vi "RTS Set Test Start Time.vi"(4 "Use Current Time As Start?":bool, 5 "Time Start (Gen Prev End)":timestamp, 6 "index":i32, 7 "Start Time Offset":dbl, 8 "Error In":errorcluster, 11 "Current Test":T1={"Chamber 1-3"=[{"End Time"=timestamp(3594046716.8947463 s since 1904-01-01), "Start Time"=timestamp(3593614713.19836 s since 1904-01-01), "Door Opening Schedule:"={"Open Door Timer (s)"=12.0, "Delay Time (s)"=695.0, "Close Door Timer (s)"=12.0}, "Enable Door Ops"=TRUE, "Door Openings"=120, "Temp (°F)"=0.0, "Humidity (%)"=0.0, "Voltage (V)"=0.0, "Door Open Sequence:"=enum."", "Door Delay(sec)"=0.0, "Dehum (°F)"=0.0, "Cool (°F)"=0.0}], "Chamber 1-2"=[{"End Time"=timestamp(3594046708.565822 s since 1904-01-01), "Start Time"=timestamp(3593614700.612354 s since 1904-01-01), "Door Opening Schedule:"={"Open Door Timer (s)"=12.0, "Delay Time (s)"=695.0, "Close Door Timer (s)"=12.0}, "Enable Door Ops"=TRUE, "Door Openings"=0, "Temp (°F)"=0.0, "Humidity (%)"=0.0, "Voltage (V)"=0.0, "Door Open Sequence:"=enum."", "Door Delay(sec)"=0.0, "Dehum (°F)"=0.0, "Cool (°F)"=0.0}], "Chamber 1-1"=[{"End Time"=timestamp(3594046691.867131 s since 1904-01-01), "Start Time"=timestamp(3593614687.850203 s since 1904-01-01), "Door Opening Schedule:"={"Open Door Timer (s)"=12.0, "Delay Time (s)"=2800.0, "Close Door Timer (s)"=12.0}, "Enable Door Ops"=TRUE, "Door Openings"=30, "Temp (°F)"=0.0, "Humidity (%)"=0.0, "Voltage (V)"=0.0, "Door Open Sequence:"=enum."", "Door Delay(sec)"=0.0, "Dehum (°F)"=0.0, "Cool (°F)"=0.0}], "Standard Tests 1-1"=enum."511-B111 Internal Moisture"} {"Chamber 1-1"."Start Time" format="%<%X\n%x>T"; "Chamber 1-1"."End Time" format="%<%X\n%x>T"; "Chamber 1-2"."Start Time" format="%<%X\n%x>T"; "Chamber 1-2"."End Time" format="%<%X\n%x>T"; "Chamber 1-3"."Start Time" format="%<%X\n%x>T"; "Chamber 1-3"."End Time" format="%<%X\n%x>T"}) -> (0 "Error Out":errorcluster, 3 "Current Test Output":T1={"Chamber 1-3"=[{"End Time"=timestamp(3594046716.8947463 s since 1904-01-01), "Start Time"=timestamp(3593614713.19836 s since 1904-01-01), "Door Opening Schedule:"={"Open Door Timer (s)"=12.0, "Delay Time (s)"=695.0, "Close Door Timer (s)"=12.0}, "Enable Door Ops"=TRUE, "Door Openings"=120, "Temp (°F)"=0.0, "Humidity (%)"=0.0, "Voltage (V)"=0.0, "Door Open Sequence:"=enum."", "Door Delay(sec)"=0.0, "Dehum (°F)"=0.0, "Cool (°F)"=0.0}], "Chamber 1-2"=[{"End Time"=timestamp(3594046708.565822 s since 1904-01-01), "Start Time"=timestamp(3593614700.612354 s since 1904-01-01), "Door Opening Schedule:"={"Open Door Timer (s)"=12.0, "Delay Time (s)"=695.0, "Close Door Timer (s)"=12.0}, "Enable Door Ops"=TRUE, "Door Openings"=0, "Temp (°F)"=0.0, "Humidity (%)"=0.0, "Voltage (V)"=0.0, "Door Open Sequence:"=enum."", "Door Delay(sec)"=0.0, "Dehum (°F)"=0.0, "Cool (°F)"=0.0}], "Chamber 1-1"=[{"End Time"=timestamp(3594046691.867131 s since 1904-01-01), "Start Time"=timestamp(3593614687.850203 s since 1904-01-01), "Door Opening Schedule:"={"Open Door Timer (s)"=12.0, "Delay Time (s)"=2800.0, "Close Door Timer (s)"=12.0}, "Enable Door Ops"=TRUE, "Door Openings"=30, "Temp (°F)"=0.0, "Humidity (%)"=0.0, "Voltage (V)"=0.0, "Door Open Sequence:"=enum."", "Door Delay(sec)"=0.0, "Dehum (°F)"=0.0, "Cool (°F)"=0.0}], "Standard Tests 1-1"=enum."511-B111 Internal Moisture"} {"Chamber 1-1"."Start Time" format="%<%X\n%x>T"; "Chamber 1-1"."End Time" format="%<%X\n%x>T"; "Chamber 1-2"."Start Time" format="%<%X\n%x>T"; "Chamber 1-2"."End Time" format="%<%X\n%x>T"; "Chamber 1-3"."Start Time" format="%<%X\n%x>T"; "Chamber 1-3"."End Time" format="%<%X\n%x>T"})   [LabVIEW 2020]
uses:
  Type Definitions/RTS Door Op Data.ctl
  Type Definitions/RTS Door Ops Client.ctl
  Type Definitions/RTS Door Opening Schedule.ctl
  Type Definitions/RTS Door Ops Sequence.ctl
  Type Definitions/RTS Standard Door Opening Test.ctl
panel:
  # "Chamber Conditions:"
  # "Chamber Conditions:"
  # "Chamber Conditions:"
  # "Chamber Conditions:"
  # "Chamber Conditions:"
  # "Chamber Conditions:"
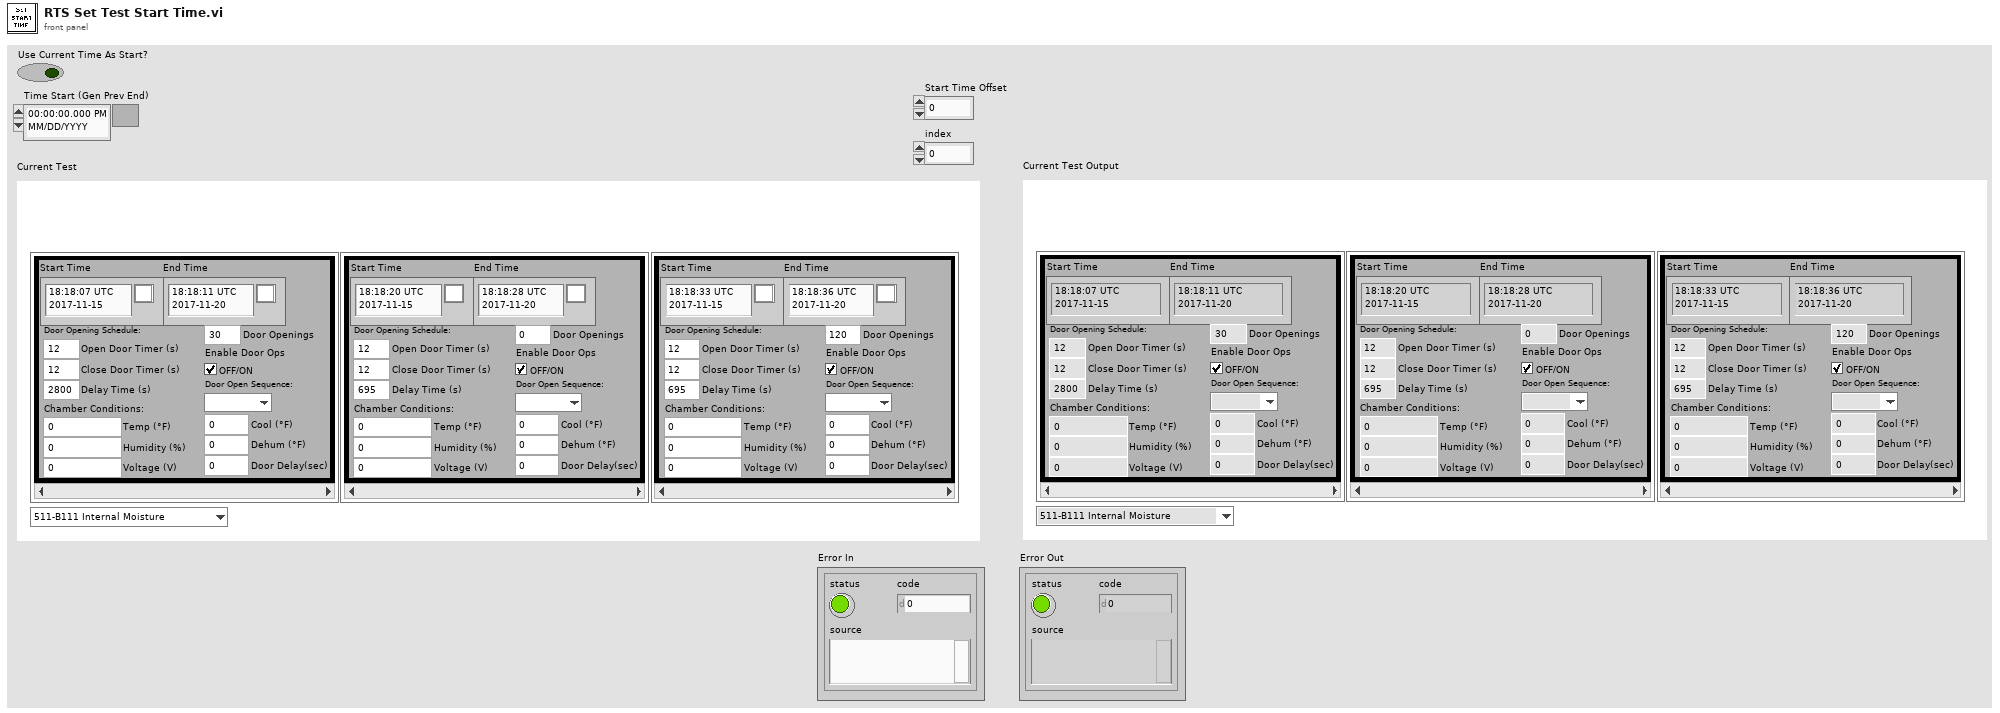
[diagram p1: front panel]
types:
  T1 = typedef "RTS Door Op Data.ctl" = cluster{"Chamber 1-3":T2[], "Chamber 1-2":T2[], "Chamber 1-1":T2[], "Standard Tests 1-1":T5}
  T2 = typedef "RTS Door Ops Client.ctl" = cluster{"End Time":timestamp, "Start Time":timestamp, "Door Opening Schedule:":T3, "Enable Door Ops":bool, "Door Openings":u32, "Temp (°F)":dbl, "Humidity (%)":dbl, "Voltage (V)":dbl, "Door Open Sequence:":T4, "Door Delay(sec)":dbl, "Dehum (°F)":dbl, "Cool (°F)":dbl}
  T3 = typedef "RTS Door Opening Schedule.ctl" = cluster{"Open Door Timer (s)":dbl, "Delay Time (s)":dbl, "Close Door Timer (s)":dbl}
  T4 = typedef "RTS Door Ops Sequence.ctl" = enum16{"", "1st", "2nd", "3rd"}
  T5 = typedef "RTS Standard Door Opening Test.ctl" = enum16{"Standard ETPs", "511-B113 EHUT", "511-B110 HUT", "512-C410 SLAT", "511-B111 Internal Moisture", "511-C401 Moisture Accumulation", "511-B100 No Door Opening (NDO)", "511-B304 ISO Energy Consumption", "Custom Test", "Cancel Test"}
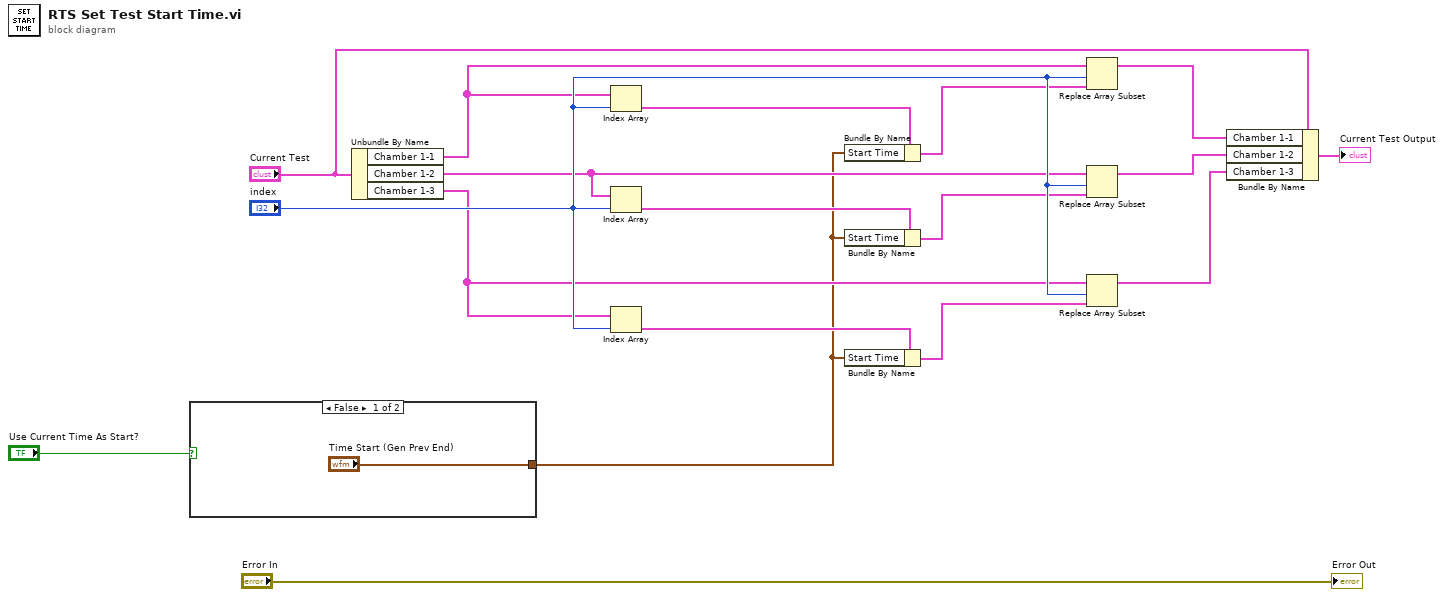
[diagram p0: block diagram]
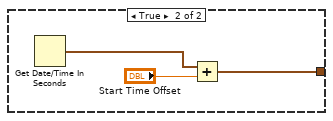
[diagram p2: hidden frame]
diagram:
  n1 = case shown="False" "Use Current Time As Start?" {
    tunnel: ["Time Start (Gen Prev End)" w20] -> w2
    frame False {
    }
    frame True {
      n2 = Get Date/Time In Seconds() -> (seconds since 1Jan1904=w22:timestamp)
      n3 = Add(x=w22, y="Start Time Offset") -> (x+y=w20:timestamp)
    }
  }
  n4 = Unbundle By Name("Current Test") -> ("Chamber 1-1"=w13:T2[], "Chamber 1-2"=w12:T2[], "Chamber 1-3"=w11:T2[])
  n5 = Index Array(array=w13, index="index") -> (element=w16:T2)
  n6 = Index Array(array=w12, index="index") -> (element=w17:T2)
  n7 = Index Array(array=w11, index="index") -> (element=w18:T2)
  n8 = Bundle By Name(cluster=w16, "Start Time"=w2) -> (w8:T2)
  n9 = Bundle By Name(cluster=w17, "Start Time"=w2) -> (w9:T2)
  n10 = Bundle By Name(cluster=w18, "Start Time"=w2) -> (w10:T2)
  n11 = Replace Array Subset(array=w13, new element=w8, index="index") -> (w6:T2[])
  n12 = Replace Array Subset(array=w12, new element=w9, index="index") -> (w5:T2[])
  n13 = Replace Array Subset(array=w11, new element=w10, index="index") -> (w4:T2[])
  n14 = Bundle By Name(cluster="Current Test", "Chamber 1-1"=w6, "Chamber 1-2"=w5, "Chamber 1-3"=w4) -> (→"Current Test Output":T1)
  "Error Out" <- "Error In"
